vi "Format Structure Table Section.vi"(8 "Error in":errorcluster caption="Error in (no error)", 11 "VI Info Array":T1[](array[typedef])) -> (0 "Error out":errorcluster, 3 "Section Text":string)   [LabVIEW 2023, in "VIDoc Printer - Confluence.lvlib" / "VIDoc Printer - Confluence.lvclass"]
uses:
  VIDoc Printer - Confluence.lvclass
  Parsing/TypeDefs/Method Spec Cluster.ctl
  Parsing/TypeDefs/VI Type Extended Enum.ctl
  <vilib>/picture/picture.llb/imagedata.ctl
  Parsing/TypeDefs/Class Dispatch Type Enum.ctl
  Parsing/TypeDefs/Controls Info Cluster.ctl
  <vilib>/Utility/miscctls.llb/LVKeyTypeDef.ctl
  <vilib>/Utility/miscctls.llb/LVPointTypeDef.ctl
  Parsing/SubVIs/Structure Reporter/Tree Cluster.ctl
  Confluence Formatting/Types/Format Combo Box.ctl
  VIDoc Printer - Confluence.lvclass/VIDoc Printer - Confluence.ctl
  Confluence Formatting/Confluence Formatting.lvlib
  <userlib>/_PetranWay/LabVIEW Confluence API/Source/PetranWay_Confluence API.lvlib
  Parsing/VIDoc Parsing.lvlib
  Parsing/SubVIs/Structure Reporter/Structure Reporter.lvlib
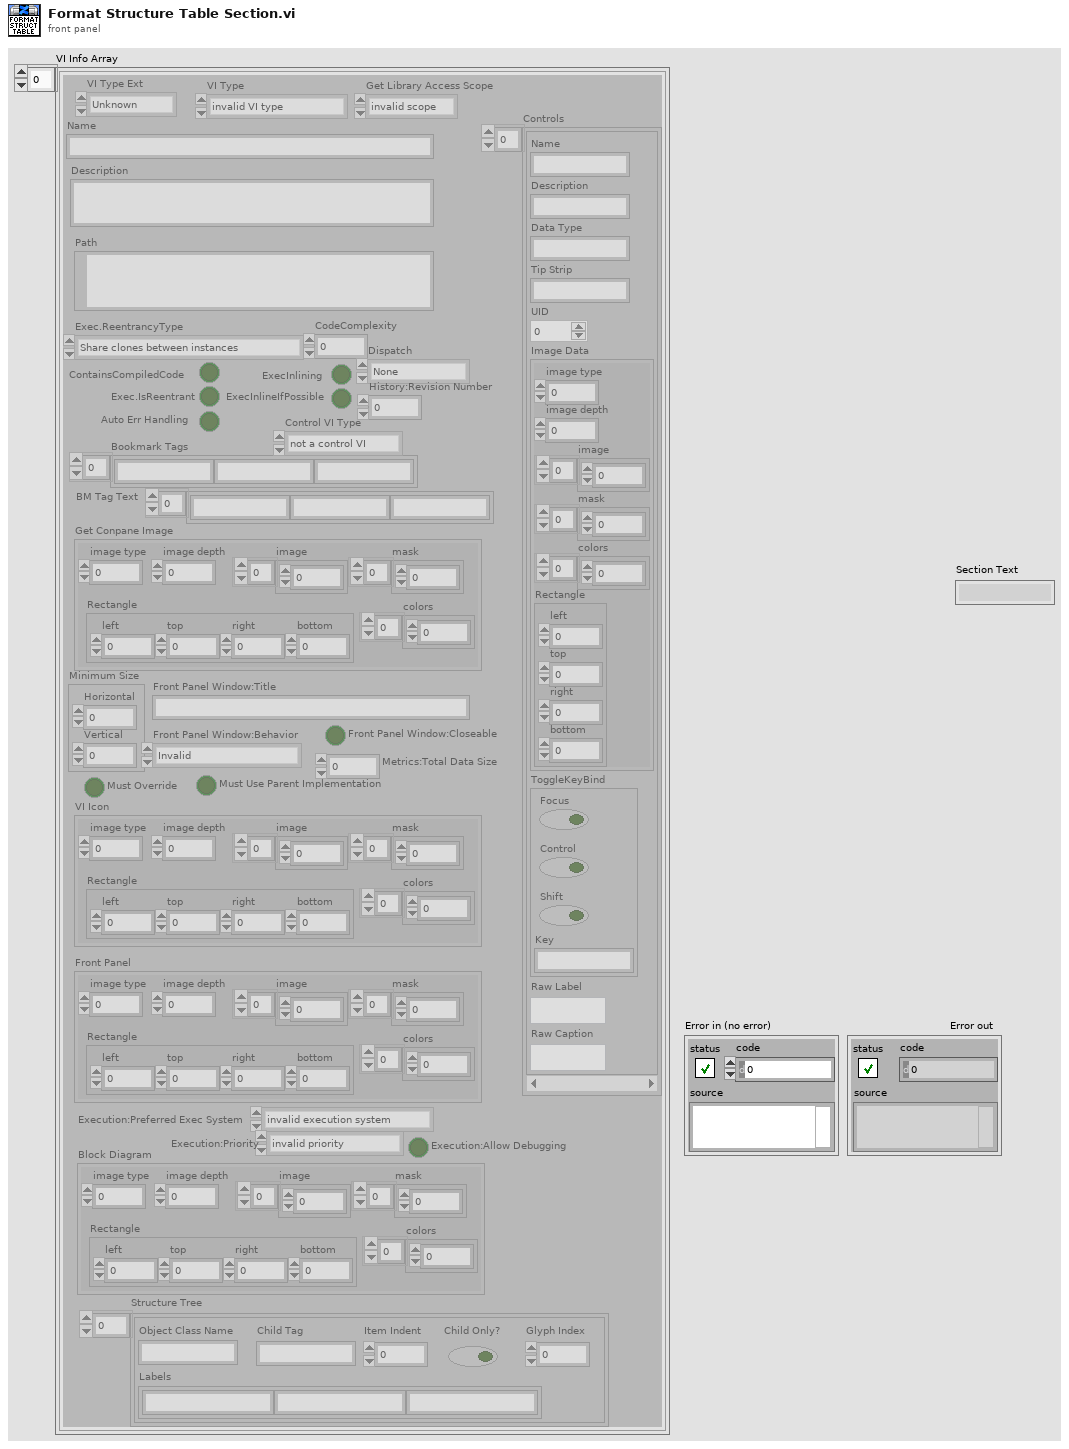
[diagram p1: front panel]
types:
  T1 = typedef "VIDoc Parsing.lvlib/Method Spec Cluster.ctl" = cluster{"VI Type Ext":T2, "Name":string, "Path":path, "Get Conpane Image":T3, "Description":string, "Get Library Access Scope":enum32{"invalid scope", "public", "private", "protected", "community"}, "Dispatch":T4, "ContainsCompiledCode":bool, "Exec.IsReentrant":bool, "Exec.ReentrancyType":enum16{"Share clones between instances", "Preallocate clone for each instance"}, "ExecInlining":bool, "ExecInlineIfPossible":bool, "Auto Err Handling":bool, "CodeComplexity":sgl, "Bookmark Tags":string[], "Control VI Type":enum32{"not a control VI", "control", "typedef", "strict typedef"}, "Controls":T5[], "VI Type":enum32{"invalid VI type", "Standard VI", "Control VI", "Global VI", "Polymorphic VI", "Configuration VI", "SubSystem", "Facade VI", "Method VI", "Statechart Diagram VI"}, "Minimum Size":T7, "Front Panel Window:Title":string, "Front Panel Window:Behavior":enum32{"Invalid", "Default", "Floating", "Floating/Auto-Hide", "Modal"}, "Front Panel Window:Closeable":bool, "Must Override":bool, "Must Use Parent Implementation":bool, "VI Icon":T3, "Front Panel":T3, "History:Revision Number":u32, "Metrics:Total Data Size":u32, "Execution:Allow Debugging":bool, "Execution:Preferred Exec System":enum32{"invalid execution system", "user interface", "standard", "instrument i/o", "data acquisition", "other 1", "other 2", "same as caller"}, "Execution:Priority":enum32{"invalid priority", "background priority", "normal priority", "above normal priority", "high priority", "time critical priority", "subroutine"}, "BM Tag Text":string[], "Block Diagram":T3, "Structure Tree":T8[]}
  T2 = typedef "VIDoc Parsing.lvlib/VI Type Extended Enum.ctl" = enum16{"Unknown", "Class Method", "Class Accessor Get", "Class Accessor Set", "Class Control", "Library Method", "Library Control", "VI", "Control"}
  T3 = typedef "imagedata.ctl" = cluster{"image type":i32, "image depth":i32, "image":u8[], "mask":u8[], "colors":u32[], "Rectangle":cluster{"left":i16, "top":i16, "right":i16, "bottom":i16}}
  T4 = typedef "VIDoc Parsing.lvlib/Class Dispatch Type Enum.ctl" = enum16{"None", "Static", "Dynamic"}
  T5 = typedef "VIDoc Parsing.lvlib/Controls Info Cluster.ctl" = cluster{"Name":string, "Description":string, "Data Type":string, "Tip Strip":string, "UID":i32, "Image Data":T3, "ToggleKeyBind":T6, "Raw Label":string, "Raw Caption":string}
  T6 = typedef "LVKeyTypeDef.ctl" = cluster{"Focus":bool, "Control":bool, "Shift":bool, "Key":string}
  T7 = typedef "LVPointTypeDef.ctl" = cluster{"Horizontal":i16, "Vertical":i16}
  T8 = typedef "VIDoc Parsing.lvlib/Structure Reporter.lvlib/Tree Cluster.ctl" = cluster{"Object Class Name":string, "Labels":string[], "Child Tag":string, "Item Indent":i32, "Child Only?":bool, "Glyph Index":i32}
  T9 = typedef "Confluence Formatting.lvlib/Format Combo Box.ctl" = string
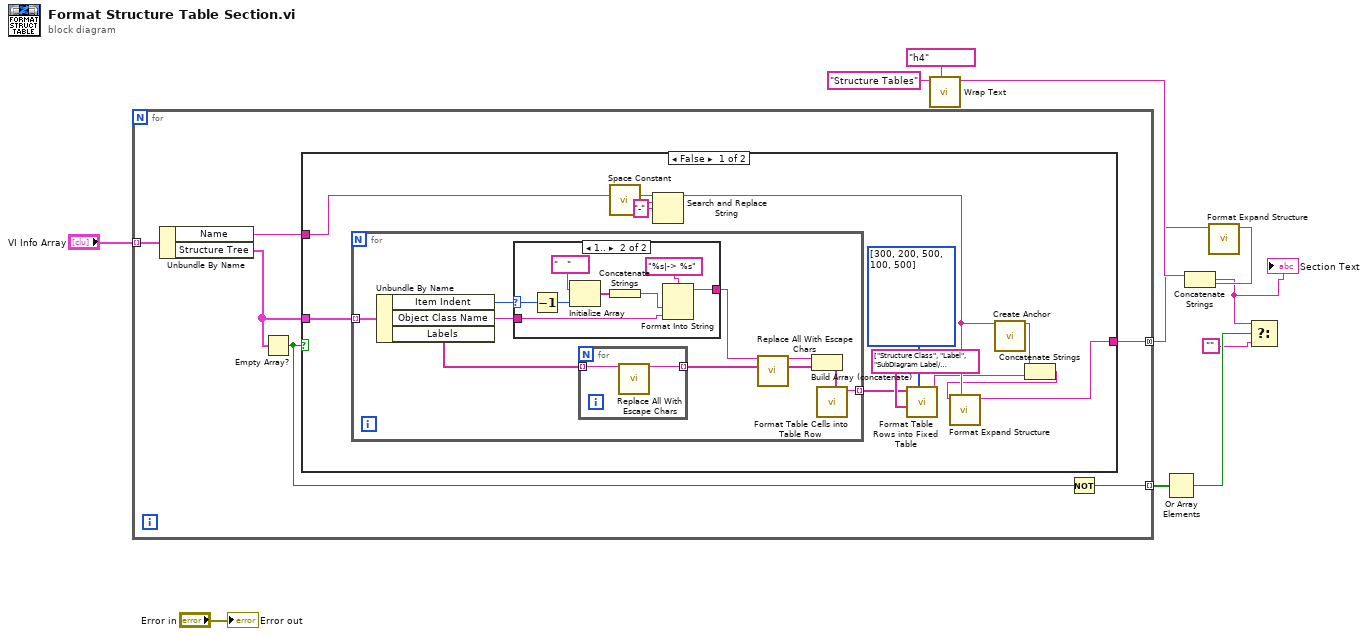
[diagram p0: block diagram]
diagram:
  n1 = for {
    tunnel: "VI Info Array" -> [w17] mode=indexing
    tunnel: [w15] -> w3 mode=concatenating
    tunnel: [w12] -> w6 mode=indexing
    n2 = Unbundle By Name(w17) -> ("Name"=w16:string, "Structure Tree"=w14:T8[])
    n3 = Empty Array?(array=w14) -> (empty?=w13:bool)
    n4 = case shown="False" w13 {
      tunnel: w14 -> [w29 _]
      tunnel: w16 -> [w22 _]
      tunnel: [w21 _] -> w15
      frame False {
        n5 = for {
          tunnel: [w38] -> w27 mode=indexing
          tunnel: w29 -> [w37] mode=indexing
          n6 = Unbundle By Name(w37) -> ("Item Indent"=w36:i32, "Object Class Name"=w35:string, "Labels"=w31:string[])
          n7 = case shown="1.." w36 {
            selector: w36 -> [_ w49]
            tunnel: w35 -> [w41 w47]
            tunnel: [w41 w46] -> w34
            frame ..0 {
            }
            frame 1.. {
              n8 = Decrement(x=w49) -> (x-1=w42:i32)
              n9 = Initialize Array("   ", w42) -> (w45:string[])
              n10 = Concatenate Strings(w45) -> (w44:string)
              n11 = Format Into String(format string="%s|-> %s", w44, w47) -> (resulting string=w46:string)  [unwired: 2 in, 1 out]
            }
          }
          n12 = for {
            tunnel: w31 -> [w40] mode=indexing
            tunnel: [w39] -> w30 mode=indexing
            n13 = call <userlib>:"Replace All With Escape Chars.vi"("Raw String"=w40) -> ("With Substitued Escape Characters"=w39:string)  [unwired: 13 in, 1 out]
          }
          n14 = call <userlib>:"Replace All With Escape Chars.vi"("Raw String"=w34) -> ("With Substitued Escape Characters"=w32:string)  [unwired: 13 in, 1 out]
          n15 = Build Array (concatenate)(w32, w30) -> (w33:string[])
          n16 = call "Format Table Cells into Table Row.vi"("Table Cells"=w33) -> ("Table Row Text"=w38:string)  [unwired: 10 in]
        }
        n17 = call <vilib>:"Space Constant.vi"() -> ("String"=w25:string)
        n18 = Search and Replace String(input string=w22, search string=w25, replace string="-" ("replace string (\"\")")) -> (result string=w23:string)  [unwired: 5 in, 3 out]
        n19 = call "Format Table Rows into Fixed Table.vi"("Column Pixel Widths"=i16[] [300, 200, 500, 100, 500], "Table Headers"=string[] ["Structure Class", "Label", "SubDiagram Label/Description", "Frame I", "Frame Condition"], "Table Rows"=w27) -> ("Table Text"=w19:string)  [unwired: 8 in]
        n20 = call <userlib>:"Create Anchor.vi"("Anchor Name"=w23) -> ("Anchor HTML"=w20:string)  [unwired: 13 in, 1 out]
        n21 = Concatenate Strings(w20, w19) -> (w18:string)
        n22 = call "Format Expand Structure.vi"("Title (Click here to expand...)"=w23, "Content"=w18) -> ("Expand String"=w21:string)  [unwired: 8 in, 1 out]
      }
      frame True {
      }
    }
    n23 = Not(x=w13) -> (.not. x?=w12:bool)
  }
  n24 = call "Wrap Text.vi"("Formatting"=T9 "h4", "String"="Structure Tables") -> ("Wrapped String"=w8:string)  [unwired: 8 in, 1 out]
  n25 = Or Array Elements(Boolean array=w6) -> (logical OR=w5:bool)
  n26 = call "Format Expand Structure.vi"("Content"=w3) -> ("Expand String"=w2:string)  [unwired: 9 in, 1 out]
  n27 = Concatenate Strings(w8, w2) -> (w1:string)
  "Section Text" <- w1
  n28 = Select(t=w1, s=w5, f="") -> ()  [unwired: 1 out]
  "Error out" <- "Error in"
